vi "task.vi"   [LabVIEW 2016, in "挥发酚.lvlib"]
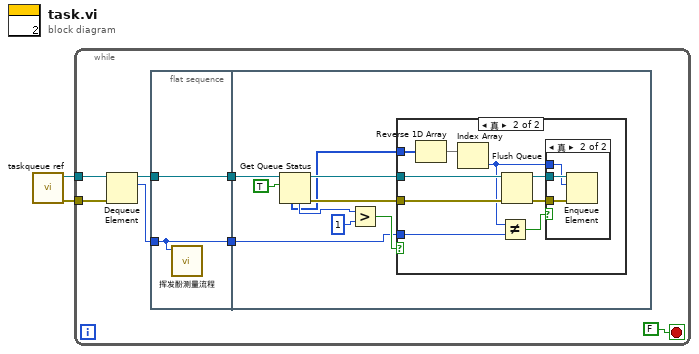
[diagram p0: block diagram]
diagram:
  n1 = call "taskqueue ref.vi"() -> ("错误输出"=w1:errorcluster, "队列输出"=w2:refnum<queue>)  [unwired: 10 in]
  n2 = while {
    tunnel: w2 -> [w9]
    tunnel: w1 -> [w8]
    stop <- FALSE stop-if-true
    n3 = Dequeue Element(queue=w9, error in (no error)=w8) -> (queue out=w7:refnum<queue>, element=w6:u16)  [unwired: 1 in, 2 out]
    n4 = flat-sequence {
      tunnel: w7 -> [w11]
      tunnel: w6 -> [w10]
      tunnel: [w11] -> w4
      tunnel: [w10] -> w3
      tunnel: w4 -> [w20]
      tunnel: w3 -> [w12]
      frame #0 {
        n5 = call "挥发酚测量流程.vi"("控制命令"=w10) -> ()  [unwired: 11 in]
      }
      frame #1 {
        n6 = Get Queue Status(queue=w20, return elements? (F)=TRUE ("返回元素？(F)")) -> (queue out=w15:refnum<queue>, error out=w14:errorcluster, # elements in queue=w18:i32, elements=w13:u16[])  [unwired: 1 in, 4 out]
        n7 = Greater?(x=w18, y=1) -> (0:w16:bool)
        n8 = case shown="真" w16 {
          tunnel: w15 -> [_ w29]
          tunnel: w14 -> [_ w28]
          tunnel: w13 -> [_ w27]
          tunnel: w12 -> [_ w22]
          frame False {
          }
          frame True {
            n9 = Reverse 1D Array(array=w27) -> (reversed array=w26:u16[])
            n10 = Index Array(array=w26) -> (element=w23:u16)  [unwired: 1 in]
            n11 = Not Equal?(x=w23, y=w22) -> (x != y?=w21:bool)
            n12 = Flush Queue(queue=w29, error in (no error)=w28) -> (queue out=w25:refnum<queue>, error out=w24:errorcluster)  [unwired: 1 out]
            n13 = case shown="真" w21 {
              tunnel: w25 -> [_ w32]
              tunnel: w24 -> [_ w31]
              tunnel: w23 -> [_ w30]
              frame False {
              }
              frame True {
                n14 = Enqueue Element(queue=w32, element=w30, error in (no error)=w31) -> ()  [unwired: 1 in, 3 out]
              }
            }
          }
        }
      }
    }
  }
